vi "Calculate Basic Statistics on Segment.vi"(9 "# of Samples Averaged\nfor standing weight\n(1000 is default)":i32, 10 "Start of Sample":i32, 11 "Dynamic Data Type":dynamicdata(waveform)) -> (0 "Minimum":dbl, 1 "Maximum":dbl, 2 "Standard Deviation":dbl, 3 "Arithmetic Mean":dbl, 4 "Range":dbl, 6 "SW Array":dbl[](array[numeric]))   [LabVIEW 2016]
panel:
  out "Waveform Chart":dbl[](graph)
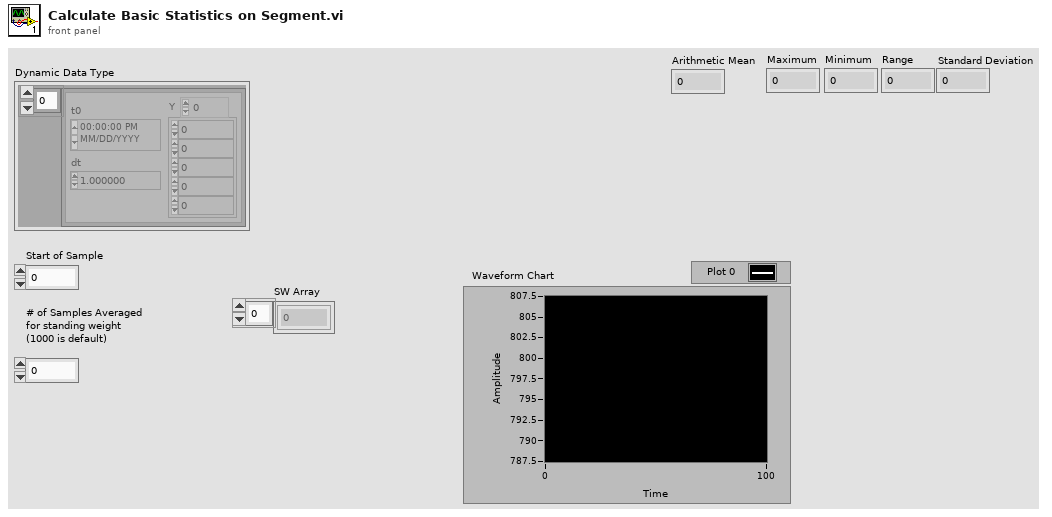
[diagram p1: front panel]
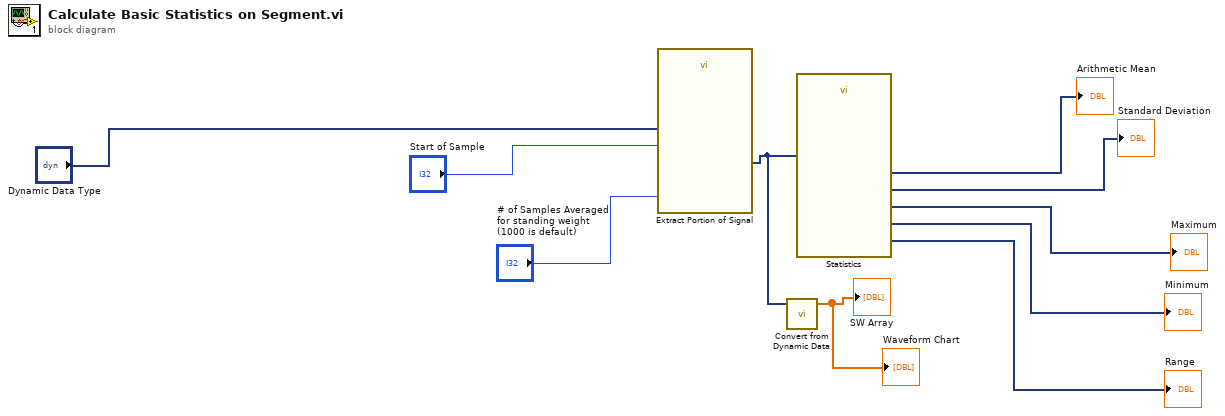
[diagram p0: block diagram]
diagram:
  n1 = call "Extract Portion of Signal"("Samples"="# of Samples Averaged\nfor standing weight\n(1000 is default)", "Begin Sample"="Start of Sample", "Signals"="Dynamic Data Type") -> ("Section"=w6:dynamicdata)  [unwired: 7 in, 1 out]
  n2 = call "Convert from Dynamic Data"("Dynamic Data Type"=w6) -> ("Array"=→"SW Array" →"Waveform Chart":dbl[])  [unwired: 3 in]
  n3 = call "Statistics"("Signals"=w6) -> ("Standard Dev"=→"Standard Deviation":dynamicdata, "Arithmetic Mean"=→"Arithmetic Mean":dynamicdata, "Range"=→"Range":dynamicdata, "Minimum"=→"Minimum":dynamicdata, "Maximum"=→"Maximum":dynamicdata)  [unwired: 21 in, 1 out]
